vi "slopes2command.vi"(8 "error in (no error)":errorcluster, 9 "HasoSlopes in":refnum<class "HasoSlopes.lvclass">, 10 "Number of kept modes":i32=52, 11 "CorrectionDataManager in":refnum<class "CorrectionDataManager.lvclass">) -> (0 "error out":errorcluster, 1 "HasoSlopes out":refnum<class "HasoSlopes.lvclass">, 2 "Offset Positions":sgl[](array[numeric]), 3 "CorrectionDataManager out":refnum<class "CorrectionDataManager.lvclass">)   [LabVIEW 2018]
uses:
  <userlib>/WaveKit.lib/Classes/CorrectionDataManager/CorrectionDataManager.lvclass
  <userlib>/WaveKit.lib/Controls/HasoSlopes.lvclass
  <userlib>/WaveKit.lib/Controls/InteractionMatrixToCommandMatrixParameters.ctl
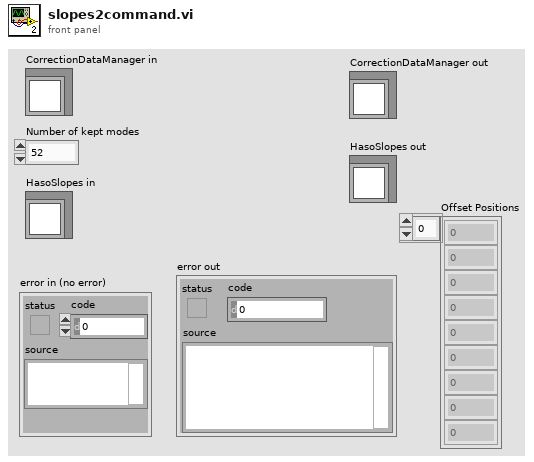
[diagram p1: front panel]
types:
  T1 = typedef "InteractionMatrixToCommandMatrixParameters.ctl" = cluster{"Number of kept modes":i32, "Tilt filtering":bool}
  T2 = typedef "Wavefront Corrector Position.ctl" = sgl[]
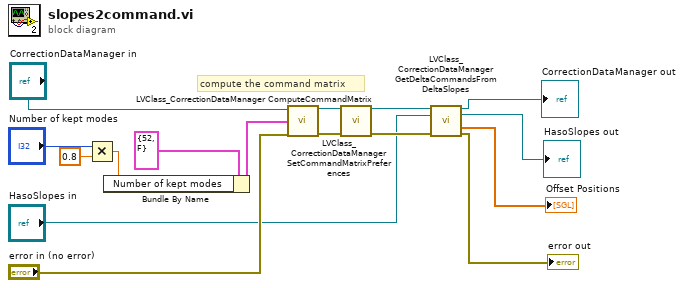
[diagram p0: block diagram]
diagram:
  # "compute the command matrix"
  n1 = Multiply(x="Number of kept modes", y=0.8) -> (x*y=w12:dbl)
  n2 = Bundle By Name(cluster=T1 {"Number of kept modes"=52, "Tilt filtering"=FALSE} ("Prefs"), "Number of kept modes"=w12) -> (w11:T1)
  n3 = call <userlib>:"LVClass_CorrectionDataManager SetCommandMatrixPreferences.vi"("CorrectionDataManager in"="CorrectionDataManager in", "Prefs"=w11, "error in (no error)"="error in (no error)") -> ("CorrectionDataManager out"=w15:refnum<class "CorrectionDataManager.lvclass">, "error out"=w10:errorcluster)  [unwired: 11 in]
  n4 = call <userlib>:"LVClass_CorrectionDataManager ComputeCommandMatrix.vi"("CorrectionDataManager in"=w15, "error in (no error)"=w10) -> ("CorrectionDataManager out"=w9:refnum<class "CorrectionDataManager.lvclass">, "error out"=w8:errorcluster)  [unwired: 12 in]
  n5 = call <userlib>:"LVClass_CorrectionDataManager GetDeltaCommandsFromDeltaSlopes.vi"("CorrectionDataManager in"=w9, "Delta Slopes IN"="HasoSlopes in", "error in (no error)"=w8) -> ("CorrectionDataManager out"=→"CorrectionDataManager out":refnum<class "CorrectionDataManager.lvclass">, "Delta Slope OUT"=→"HasoSlopes out":refnum<class "HasoSlopes.lvclass">, "DeltaPosition"=→"Offset Positions":T2, "error out"=→"error out":errorcluster)  [unwired: 8 in, 1 out]
